vi "N06_Parallell_Loops_Variable.vi"() -> ()   [LabVIEW 2023]
panel:
  out "Local Write Loop":dbl
  out "Local Read Loop":dbl
  in  "Local Set":dbl
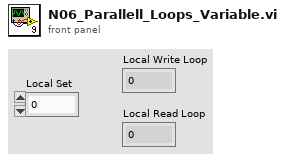
[diagram p1: front panel]
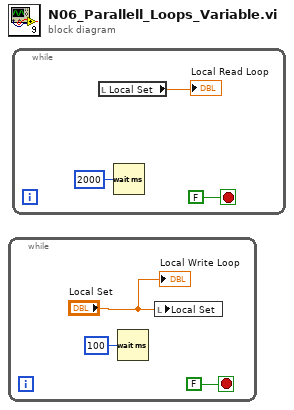
[diagram p0: block diagram]
diagram:
  n1 = while {
    stop <- FALSE stop-if-true
    n2 = Wait (ms)(milliseconds to wait=u32 100) -> ()  [unwired: 1 out]
    n3 = local write "Local Set"("Local Set") -> ()
    "Local Write Loop" <- "Local Set"
  }
  n4 = while {
    stop <- FALSE stop-if-true
    n5 = local read "Local Set"() -> (→"Local Read Loop":dbl)
    n6 = Wait (ms)(milliseconds to wait=u32 2000) -> ()  [unwired: 1 out]
  }
